vi "tearDown.vi"(8 "error in (no error)":errorcluster, 11 "reference in":refnum<class "Acyclic Logging Loopback.lvclass">) -> (0 "error out":errorcluster, 3 "reference out":refnum<class "Acyclic Logging Loopback.lvclass">)   [LabVIEW 2020, in "Acyclic Logging Loopback.lvclass"]
doc: "tearDown runs after the test method has completed. Use this method to clean up any operations or references that were opened by setUp or the test method. Unit tests should be independent of other unit tests so this VI should ensure that the next test can run in a 'clean' test environment."
uses:
  Acyclic Logging Loopback.lvclass
  Acyclic Logging Loopback.lvclass/Acyclic Logging Loopback.ctl
  <vilib>/WebDAVClient/NI_WebDAV.lvlib
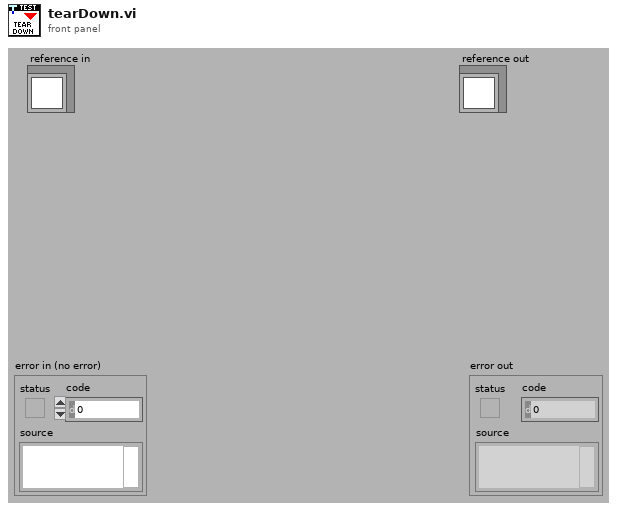
[diagram p1: front panel]
types:
  T1 = typedef "NI_WebDAV.lvlib/SessionHandle.ctl" = refnum<k1>
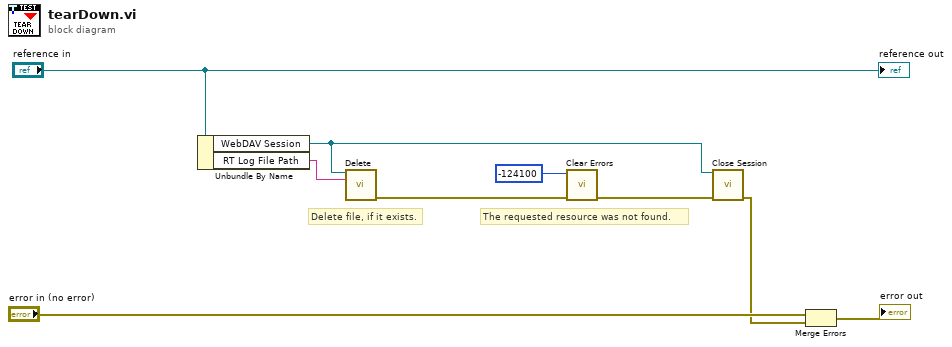
[diagram p0: block diagram]
diagram:
  # "Delete file, if it exists."
  # "The requested resource was not found."
  n1 = Unbundle By Name("reference in") -> ("WebDAV Session"=w2:T1, "RT Log File Path"=w4:string)
  n2 = call <vilib>:"Delete.vi"("session handle"=w2, "relative uri"=w4) -> ("error out"=w6:errorcluster)  [unwired: 12 in, 1 out]
  n3 = call <vilib>:"Clear Errors.vi"("error in (no error)"=w6, "specific error code to clear (0: all)"=-124100) -> ("error out"=w3:errorcluster)  [unwired: 4 in, 1 out]
  n4 = call <vilib>:"Close Session.vi"("session handle"=w2, "error in (no error)"=w3) -> ("error out"=w1:errorcluster)  [unwired: 13 in]
  n5 = Merge Errors("error in (no error)", w1) -> (→"error out":errorcluster)
  "reference out" <- "reference in"
